vi "Add One Car.vi"(8 "error in (no error)":errorcluster, 10 "Driving":bool, 11 "Zone in":refnum<class "Zone.lvclass">) -> (0 "error out":errorcluster, 3 "Zone out":refnum<class "Zone.lvclass">)   [LabVIEW 2017, in "Zone.lvclass"]
uses:
  Zone.lvclass
  Zone.lvclass/Zone.ctl
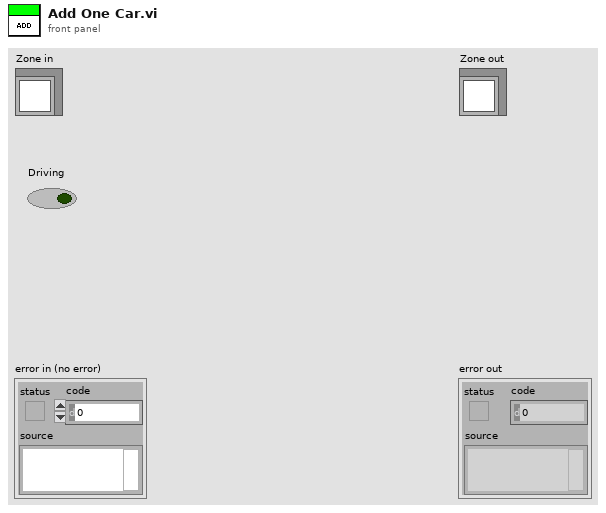
[diagram p1: front panel]
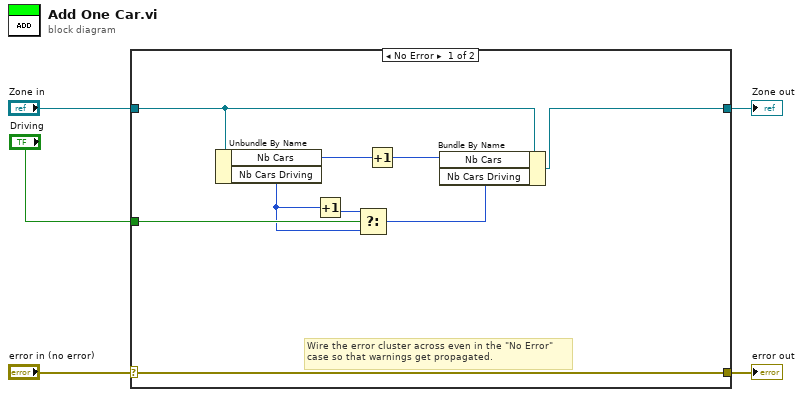
[diagram p0: block diagram]
diagram:
  n1 = case shown="No Error" "error in (no error)" {
    selector: "error in (no error)" -> [w14 w16]
    tunnel: [w14 w16] -> w4
    tunnel: [w12 w15] -> w2
    tunnel: "Zone in" -> [w13 w15]
    tunnel: "Driving" -> [w9 _]
    frame No Error {
      # "Wire the error cluster across even in the \"No Error\"\ncase so that warnings get propagated."
      n2 = Unbundle By Name(w13) -> ("Nb Cars"=w11:u32, "Nb Cars Driving"=w8:u32)
      n3 = Increment(x=w8) -> (x+1=w7:u32)
      n4 = Select(t=w7, s=w9, f=w8) -> (s? t:f=w6:u32)
      n5 = Increment(x=w11) -> (x+1=w10:u32)
      n6 = Bundle By Name(cluster=w13, "Nb Cars"=w10, "Nb Cars Driving"=w6) -> (w12:refnum<class "Zone.lvclass">)
    }
    frame Error {
    }
  }
  "error out" <- w4
  "Zone out" <- w2
